vi "Move DC_1_Distance.vi"(0 "NXT":T1, 1 "DC Motor":cluster{"DC Motor":T2, "Address":i16}={"DC Motor"=enum."DC Motor", "Address"=-1}, 2 "Return Mode (When Move Completes)":u16(ring) items=["When Move Completes", "Immediately"], 3 "Timeout (2.5 sec)":sgl=2.5, 5 "Encoder Counts":i32=100, 7 "Speed (100)":i8=100) -> (4 "NXT":T1)   [LabVIEW 2012, in "4134Outputs.lvlib"]
uses:
  4134Outputs.lvlib
  <vilib>/NXT/Subs/MotorXNode.DC Motor Type.ctl
  <vilib>/NXT/Subs/LVHSConnector.ctl
  <vilib>/NXT/LegoClasses/BrickReference/BrickReference.lvclass
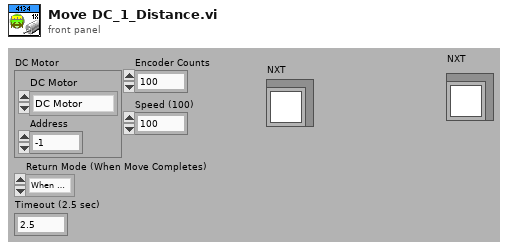
[diagram p1: front panel]
types:
  T1 = typedef "LVHSConnector.ctl" = refnum<class "BrickReference.lvclass">
  T2 = typedef "MotorXNode.DC Motor Type.ctl" = enum16{"DC Motor"}
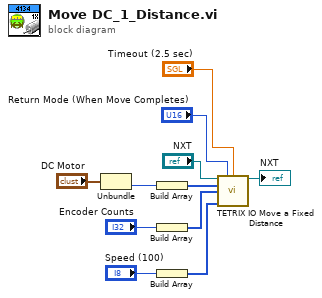
[diagram p0: block diagram]
diagram:
  n1 = Unbundle("DC Motor") -> ("Address"=w10:i16)  [unwired: 1 out]
  n2 = Build Array(w10) -> (w1:i16[])
  n3 = Build Array("Encoder Counts") -> (w5:i32[])
  n4 = Build Array("Speed (100)") -> (w4:i8[])
  n5 = call <vilib>:"TETRIX IO Move a Fixed Distance.vi"("NXT"="NXT", "VI Returns (When Move Completes)"="Return Mode (When Move Completes)", "Timeout (2.5 sec)"="Timeout (2.5 sec)", "DC Motors"=w1, "Encoder Counts"=w5, "Speed (0)"=w4) -> ("NXT"=→"NXT":T1)  [unwired: 9 in]
